vi "PutNegativeFixedInt.vi"(8 "error in (no error)":errorcluster, 10 "Number":i8, 11 "MsgPackSerializer in":refnum<class "MsgPackSerializer.lvclass">) -> (0 "error out":errorcluster, 3 "MsgPackSerializer out":refnum<class "MsgPackSerializer.lvclass">)   [LabVIEW 2015, in "MsgPackSerializer.lvclass"]
uses:
  MsgPackSerializer.lvclass
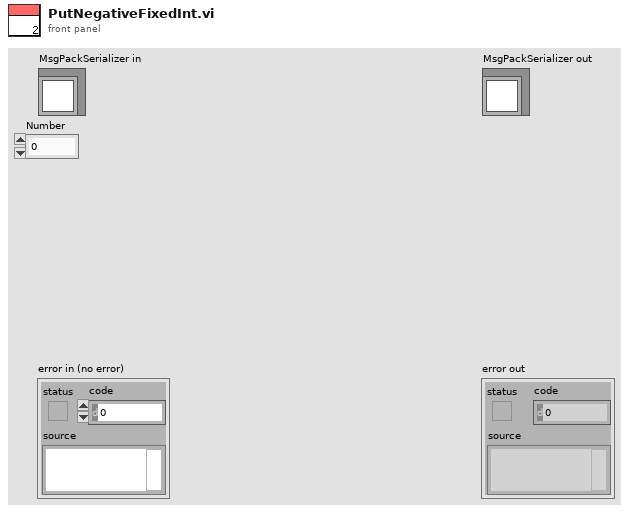
[diagram p1: front panel]
types:
  T1 = enum16{"big-endian, network order", "native, host order", "little-endian"}
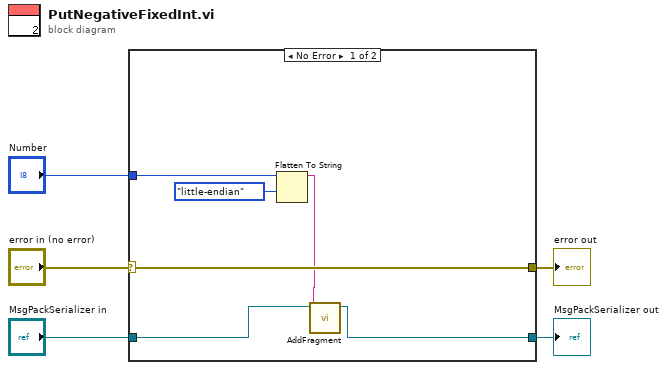
[diagram p0: block diagram]
diagram:
  n1 = case shown="No Error" "error in (no error)" {
    selector: "error in (no error)" -> [w11 w13]
    tunnel: [w11 w13] -> w4
    tunnel: [w8 w12] -> w2
    tunnel: "MsgPackSerializer in" -> [w9 w12]
    tunnel: "Number" -> [w6 _]
    frame No Error {
      n2 = Flatten To String(anything=w6, byte order (0:big-endian, network order)=T1."little-endian") -> (data string=w7:string)  [unwired: 2 in, 2 out]
      n3 = call "AddFragment.vi"("Fragment"=w7, "MsgPackSerializer in"=w9) -> ("MsgPackSerializer out"=w8:refnum<class "MsgPackSerializer.lvclass">)  [unwired: 8 in, 1 out]
    }
    frame Error {
    }
  }
  "error out" <- w4
  "MsgPackSerializer out" <- w2
